vi "IMUtoNormalGyro.vi"(1 "IMUAxis":dbl) -> (0 "NormalValue":i32)   [LabVIEW 2015]
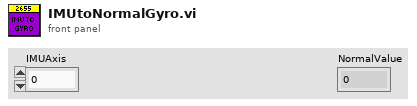
[diagram p1: front panel]
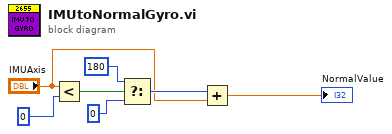
[diagram p0: block diagram]
diagram:
  n1 = Less?(x="IMUAxis", y=0) -> (x < y?=w7:bool)
  n2 = Select(t=180, s=w7, f=0) -> (s? t:f=w3:i32)
  n3 = Add(x=w3, y="IMUAxis") -> (x+y=→"NormalValue":dbl)
